vi "OFDM_Demodulation.vi"(10 "Frequency channel estimation":cdb[](array[numeric]) format="%.2f", 11 "Input sequence":cdb[](array[numeric])) -> (3 "Output sequence":cdb[](array[numeric]))   [LabVIEW 2014]
uses:
  <vilib>/Analysis/2dsp.llb/Complex FFT.vi
  <vilib>/Analysis/baseanly.llb/Mean (CDB).vi
  <vilib>/Analysis/NI_AALPro.lvlib
  <vilib>/Analysis/NI_AALBase.lvlib
panel:
  out "x/y":cdb[](array[numeric])
  out "Waveform Graph":dbl[](graph)
  out "size(s)":i32
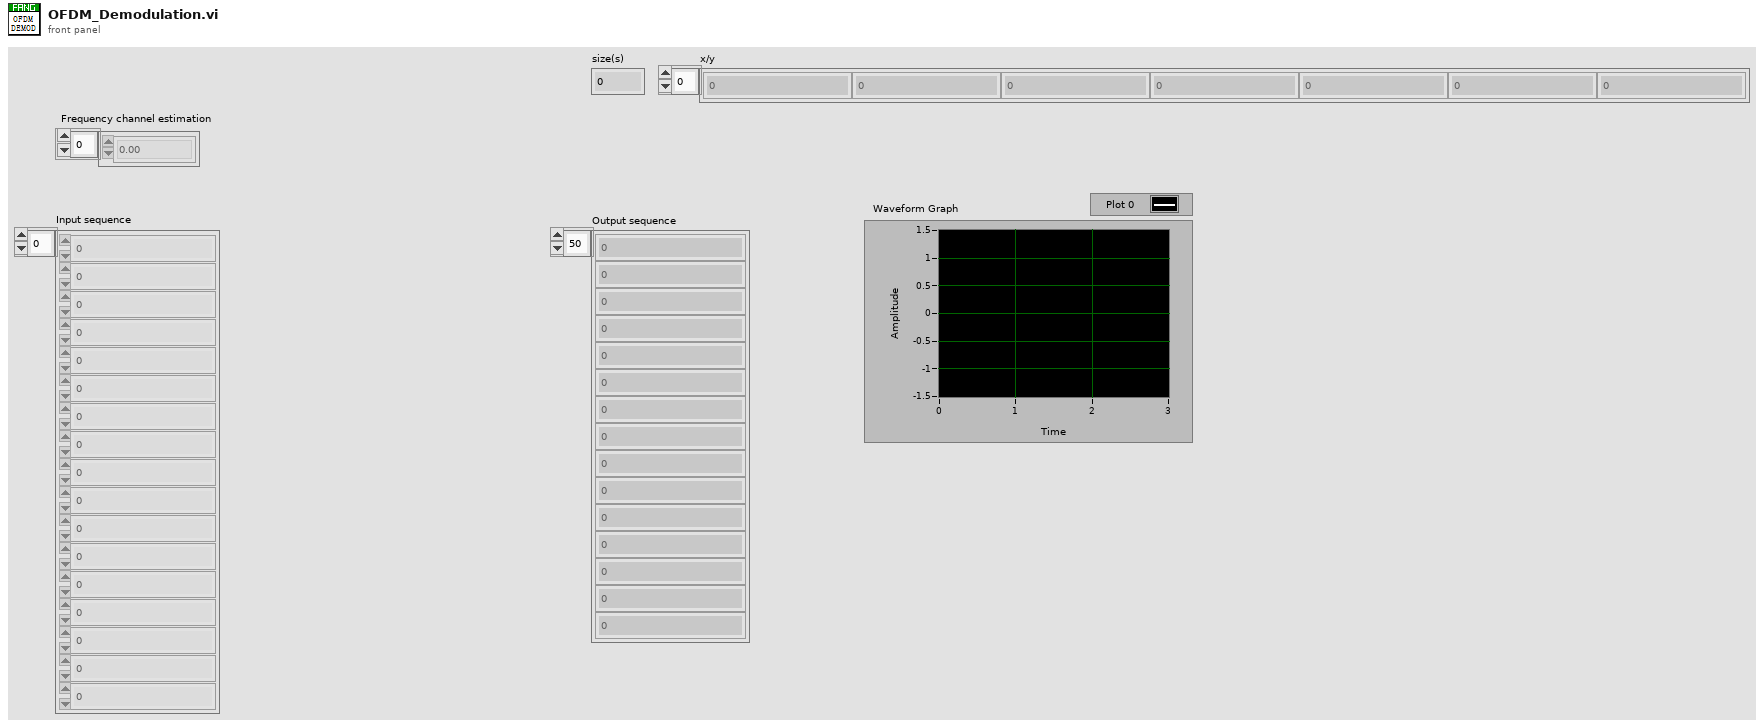
[diagram p1: front panel]
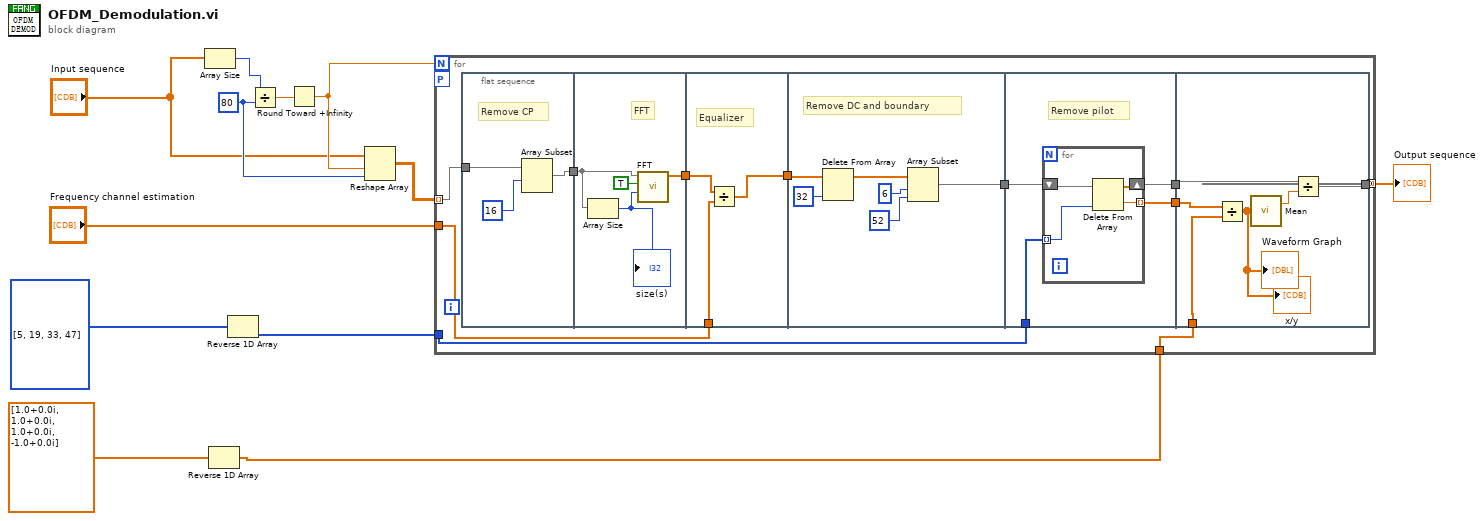
[diagram p0: block diagram]
diagram:
  w8 = 80 ("y")
  n1 = Array Size(array="Input sequence") -> (size(s)=w12:i32)
  n2 = Reverse 1D Array(array=cdb[] [1.0+0.0i, 1.0+0.0i, 1.0+0.0i, -1.0+0.0i]) -> (reversed array=w1:cdb[])
  n3 = Reverse 1D Array(array=i32[] [5, 19, 33, 47]) -> (reversed array=w6:i32[])
  n4 = Divide(x=w12, y=w8) -> (x/y=w11:dbl)
  n5 = Round Toward +Infinity(x=w11) -> (ceil(x): smallest int >= x=w9:dbl)
  n6 = Reshape Array("Input sequence", w9, w8) -> (w10:cdb[][])
  n7 = for {
    N: w9 -> [_]
    tunnel: w10 -> [w21] mode=indexing
    tunnel: w6 -> [w22]
    tunnel: [w16] -> w5 mode=concatenating
    tunnel: "Frequency channel estimation" -> [w18]
    tunnel: w1 -> [w13]
    workers-P: _ -> [_]
    n8 = flat-sequence {
      tunnel: w21 -> [w26]
      tunnel: [w24] -> w19
      tunnel: [w28] -> w20
      tunnel: w19 -> [w27]
      tunnel: w20 -> [w32]
      tunnel: w18 -> [w33]
      tunnel: [w31] -> w17
      tunnel: [w34] -> w23
      tunnel: w17 -> [w37]
      tunnel: w23 -> [w43]
      tunnel: w22 -> [w42]
      tunnel: [w41] -> w15
      tunnel: [w40] -> w14
      tunnel: [w50] -> w16
      tunnel: w15 -> [w51]
      tunnel: w14 -> [w49]
      tunnel: w13 -> [w53]
      frame #0 {
        # "Remove CP"
        n9 = Array Subset(array=w26, index=16) -> (w24:cdb[])  [unwired: 1 in]
      }
      frame #1 {
        # "FFT"
        n10 = Array Size(array=w27) -> (size(s)=w29:i32)
        "size(s)" <- w29
        n11 = call-poly <vilib>:"FFT.vi"("FFT size"=w29, "shift?"=TRUE, "X"=w27) -> ("FFT {X}"=w28:cdb[])  [unwired: 7 in, 1 out]
      }
      frame #2 {
        # "Equalizer"
        n12 = Divide(x=w32, y=w33) -> (x/y=w31:cdb[])
      }
      frame #3 {
        # "Remove DC and boundary"
        n13 = Delete From Array(array=w37, index=32) -> (array with subset deleted=w35:cdb[])  [unwired: 1 in, 1 out]
        n14 = Array Subset(array=w35, index=6, length=52) -> (w34:cdb[])
      }
      frame #4 {
        # "Remove pilot"
        n15 = for {
          shift-right: [w47] -> w41
          shift-left: w43 -> [w46]
          tunnel: w42 -> [w45] mode=indexing
          tunnel: [w44] -> w40 mode=indexing
          n16 = Delete From Array(array=w46, index=w45) -> (deleted portion=w44:cdb, array with subset deleted=w47:cdb[])  [unwired: 1 in]
        }
      }
      frame #5 {
        n17 = Divide(x=w49, y=w53) -> (x/y=w48:cdb[])
        "Waveform Graph" <- w48
        "x/y" <- w48
        n18 = call-poly <vilib>:"Mean.vi"("X"=w48) -> ("mean"=w52:cdb)  [unwired: 1 out]
        n19 = Divide(x=w51, y=w52) -> (x/y=w50:cdb[])
      }
    }
  }
  "Output sequence" <- w5
